vi "salvaexel.vi"(2 "appended array":string[][](array[string]), 3 "file name p/ exell":string) -> (0 "spreadsheet string":string)   [LabVIEW 2018]
doc: "Esta VI salva numeros reais de duas dimensoes em um arquivo com caminho especificado."
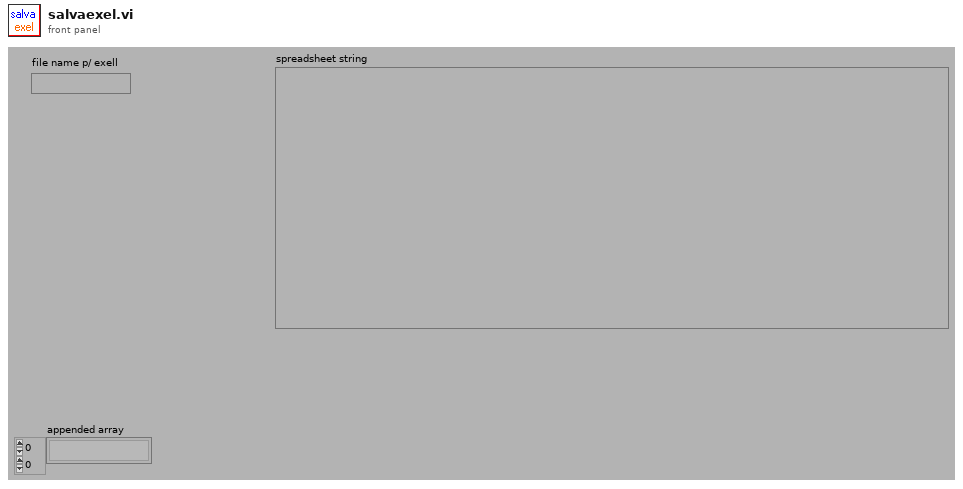
[diagram p1: front panel]
types:
  T1 = enum16{"open", "open or create", "create or replace", "create"}
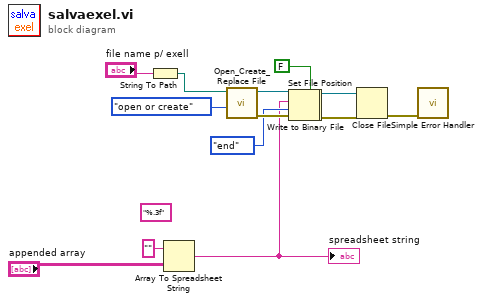
[diagram p0: block diagram]
diagram:
  (unwired) "%.3f" ("format string")
  n1 = String To Path(string="file name p/ exell") -> (path=w7:path)
  n2 = Array To Spreadsheet String(array="appended array", 3:"" ("format string")) -> (spreadsheet string=w8:string)  [unwired: 1 in]
  "spreadsheet string" <- w8
  n3 = call <vilib>:"Open_Create_Replace File.vi"("function (open:0)"=T1."open or create", "file path"=w7) -> ("error out"=w11:errorcluster, "refnum"=w14:refnum<file>)  [unwired: 6 in, 2 out]
  n4 = Set File Position(refnum=w14, from (0:start)=enum16{"start", "end", "current"}."end" ("pos mode (0:2)"), error in=w11) -> (refnum out=w3:refnum<file>, error out=w2:errorcluster)  [unwired: 1 in]
  n5 = Write to Binary File(file (use dialog)=w3, data=w8, error in=w2, 5:FALSE ("prepend array or string size? (T)")) -> (refnum out=w13:refnum<file>, error out=w12:errorcluster)  [unwired: 2 in, 1 out]
  n6 = Close File(refnum=w13, error in=w12) -> (error out=w15:errorcluster)  [unwired: 1 out]
  n7 = call <vilib>:"Simple Error Handler.vi"("error in (no error)"=w15) -> ()  [unwired: 4 in, 5 out]
